vi "Teleop.vi"(10 "Match Info":T4={"Autonomous Elapsed Seconds"=0.0, "TeleOp Elapsed Seconds"=0.0, "Disabled Elapsed Seconds"=0.0, "Visited Autonomous"=FALSE, "Visited TeleOp"=FALSE, "Visited Disabled"=FALSE, "Autonomous Settings"={"Autonomous Style"=enum."Independent", "VI Refnum"=refnum}}, 11 "Call Context":T5) -> ()   [LabVIEW 2018]
doc: "This VI is called for each TeleOp packet received from the DS where the robot is not disabled. It is often used to read from the joysticks and update I/O or to update setpoints for timed control loops. It should complete and return within 20 milliseconds or it may miss DS packets."
uses:
  <vilib>/Rock Robotics/WPI/DriverStation/WPI_DriverStationDerivedRobotMode.ctl
  <vilib>/Rock Robotics/WPI/DriverStation/WPI_DriverStationMatch Info.ctl
  <vilib>/Rock Robotics/WPI/Solenoid/WPI_SolenoidValue.ctl
  <vilib>/Rock Robotics/WPI/ThirdParty/Phoenix-LabVIEW/Motor Controller/Controls/CTRE_Phoenix_MotorControl_ControlMode.ctl
  <vilib>/Rock Robotics/WPI/Utilities/WPI_GetSetVariantRefNum.vi
  <vilib>/Rock Robotics/WPI/Joystick/WPI_JoystickArcadeMapping.vi
  <vilib>/Rock Robotics/Network Tables/NT Write Boolean Array.vi
  <vilib>/Rock Robotics/Network Tables/NT Write Numeric Array.vi
  <vilib>/Rock Robotics/WPI/Solenoid/WPI_SolenoidSetEnum.vi
  <vilib>/Rock Robotics/WPI/ThirdParty/Phoenix-LabVIEW/Motor Controller/Get/CTRE_Phoenix_MotorController_GetSelectedSensorData.vi
  <vilib>/Rock Robotics/Network Tables/NT Read Boolean.vi
  Toolbox/Simple Limit Switch/Limits(Switch+Encoder).vi
  Toolbox/Simple Limit Switch/Limits(DoubleSwitch).vi
  Toolbox/Simple Limit Switch/Limits(SingleSwitch).vi
  <vilib>/Rock Robotics/Network Tables/NT Write Number.vi
panel:
  in  "Wrist Setpoints":dbl[](array[numeric])=[-144418.0, -146243.0, -22471.0, -33508.0, -1418.0, -92418.0, -108418.0, -72418.0, -202418.0]
  in  "Positive Feeder":dbl=1.0
  in  "Negative Feeder":dbl=-0.5
  out "Wrist  Encoder Value":i32
  out "Wrist Out":dbl
  out "Wrist PID Out":dbl
  out "Elevator Out":dbl
  out "Elevator PID Out":dbl
  in  "Outer Invert Motor Limit":bool
  in  "Outer Invert Encoder Limit":bool=TRUE
  in  "Outer Limit":dbl format="%#_13g"
  in  "Horse Invert Encoder Limit":bool=TRUE
  in  "Wrist Invert Encoder Limit":bool=TRUE
  in  "Elevator Invert Encoder Limit":bool=TRUE
  out "Horse Limit Switch":bool
  in  "Reset Horse Encoder":bool
  out "OuterStageSwitch":bool
  out "Wrist After Dangerzone":T1(ring)
  out "Elevator  After Dangerzone":T2(ring)
  in  "Elevator Auto":bool=TRUE
  in  "Elevator Output Range":cluster{"output high":dbl, "output low":dbl}={"output high"=0.66176470588, "output low"=-0.75}
  in  "Elevator PID Gains":T3={"proportional gain (Kc)"=-1e-05, "integral time (Ti, min)"=0.0, "derivative time (Td, min)"=0.0}
  in  "Elevator Setpoints":dbl[](array[numeric])=[-10000.0, -10000.0, -10000.0, 405000.0, 405000.0, -10000.0]
  in  "Wrist Auto":bool=TRUE
  in  "Wrist Output Range":cluster{"output high":dbl, "output low":dbl}={"output high"=0.5, "output low"=-0.5}
  in  "Wrist PID Gains":T3={"proportional gain (Kc)"=6e-05, "integral time (Ti, min)"=0.0, "derivative time (Td, min)"=0.0}
  in  "Wrist Invert Motor Limit":bool=TRUE
  out "Wrist Limit Switch":bool
  out "Elevator Limit Switch Top":bool
  in  "Elevator Invert Motor Limit":bool=TRUE
  in  "Intake Encoder Limit":dbl=-130000.0 format="%#_13g"
  in  "Intake Home Encoder Limit":dbl=-45000.0 format="%#_13g"
  in  "HorseDanger":i32=-600000
  in  "Horse  Encoder Limit":dbl=-190000.0 format="%#_13g"
  in  "Horse Invert Motor Limit":bool=TRUE
  out "Elevator Limit Switch":bool
  out "Elevator Encoder":i32=-47
  in  "Reset Elevator Encoder":bool
  out "Horse Encoder":i32
  in  "Reset Wrist Encoder":bool
  out "Intake Wrist Encoder":i32
  # "BETA POWER/DIRECTIONS\nElevator: Negative is up\nHorse: Negative is into robot\nOuter: Positive is down\nWrist: Negative is into robot"
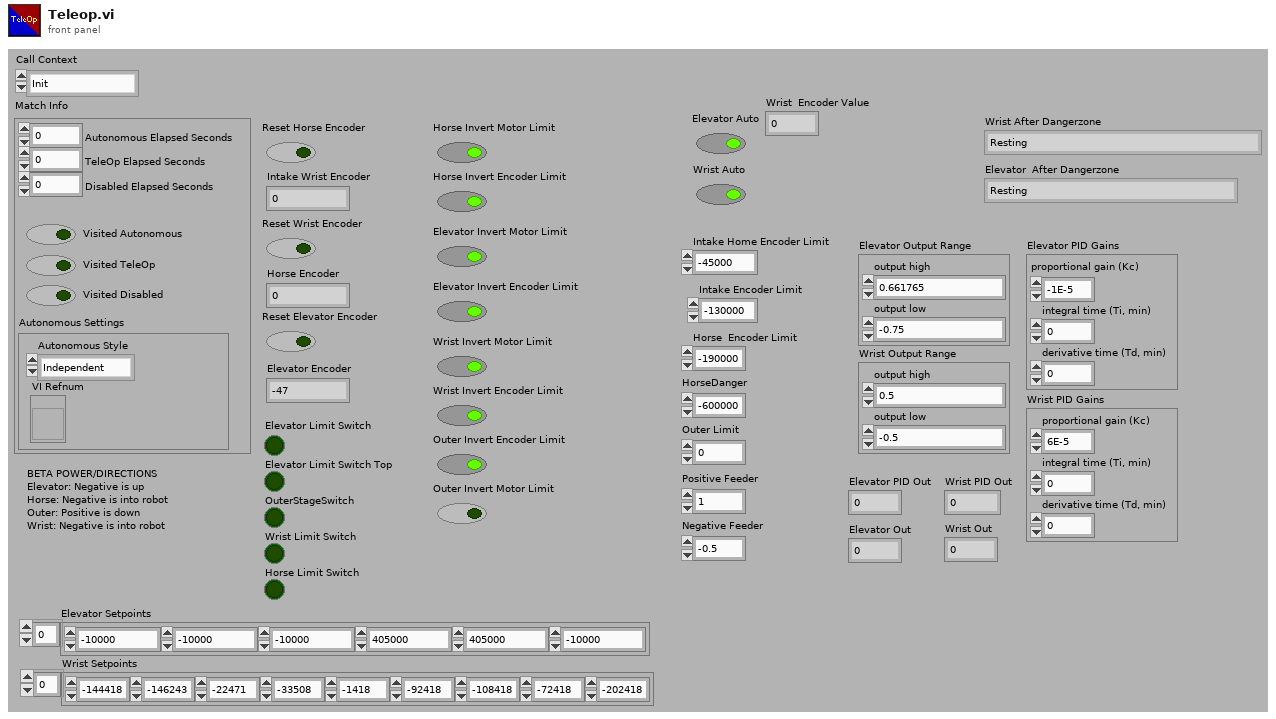
[diagram p1: front panel]
types:
  T1 = enum16{"Resting", "Hatch Ground Intake", "Hatch Place Low/Mid/CargoShip", "Hatch Place High", "Cargo Ground Intake", "Cargo Place Low/Mid", "Cargo Place High", "CargoShip Place Front", "CargoShip Place Back"}
  T2 = enum16{"Resting", "CargoShip Front", "CargoShip Back", "Cargo Mid", "Hatch Mid", "All High"}
  T3 = cluster{"proportional gain (Kc)":dbl, "integral time (Ti, min)":dbl, "derivative time (Td, min)":dbl}
  T4 = typedef "WPI_DriverStationMatch Info.ctl" = cluster{"Autonomous Elapsed Seconds":dbl, "TeleOp Elapsed Seconds":dbl, "Disabled Elapsed Seconds":dbl, "Visited Autonomous":bool, "Visited TeleOp":bool, "Visited Disabled":bool, "Autonomous Settings":cluster{"Autonomous Style":enum16{"Iterative", "Independent"}, "VI Refnum":refnum<vi>}}
  T5 = typedef "WPI_DriverStationDerivedRobotMode.ctl" = enum16{"Init", "Execute", "Stop"}
  T6 = typedef "WPI_SolenoidValue.ctl" = enum16{"Off", "On", "Forward", "Reverse"}
  T7 = enum16{"Intake Cargo", "Outtake Cargo", "Resting Cargo", "Intake Hatches", "Outtake Hatches", "Resting Hatches"}
  T8 = enum16{"Elevator Level 1", "Elevator Level 2", "Elevator Level 3"}
  T9 = typedef "CTRE_Phoenix_MotorControl_ControlMode.ctl" = u16
  T10 = cluster{"Intake Wheels Forwards":bool, "Elevator Shift":bool, "Intake Wheels Backwards":bool, "Drivetrain Shift":bool, "Elevator Outer Forwards":bool, "Elevator Outer Backwards":bool, "Hatch Telescope":bool, "Hatch Intake Clamp":bool, "Horse Drive Up":bool, "Horse Drive Down":bool, "Level 3 Climb":bool}
  T11 = typedef "WPI_JoystickDevRef.ctl" = cluster{"Device":T12}
  T12 = typedef "WPI_JoystickDeviceEnum.ctl" = enum16{"USB 0", "USB 1", "USB 2", "USB 3", "USB 4", "USB 5"}
  T13 = typedef "WPI_MotorControlDeviceRef.ctl" = cluster{"DeviceStatus":errorcluster, "Type":T14, "PWM":cluster{"PWM Channel":T15, "DeadBand":T16}, "CAN":cluster{"Device Number":u8, "SetOutput VI Ref":variant, "GetOutput VI Ref":variant, "Enable VI Ref":variant, "Disable VI Ref":variant, "Data":variant}, "Invert":bool, "DIO PWM":cluster{"PWM \"Enable\" Channel":T15, "DIOChannel":T17, "PWM Rate":dbl}}
  T14 = typedef "WPI_MotorControlType.ctl" = enum16{"PWM", "CAN", "DIO PWM"}
  T15 = typedef "FPGA_DIOPWMChannel.ctl" = enum8{"PWM 0", "PWM 1", "PWM 2", "PWM 3", "PWM 4", "PWM 5", "PWM 6", "PWM 7", "PWM 8", "PWM 9", "PWM MXP 0", "PWM MXP 1", "PWM MXP 2", "PWM MXP 3", "PWM MXP 4", "PWM MXP 5", "PWM MXP 6", "PWM MXP 7", "PWM MXP 8", "PWM MXP 9", "Invalid"}
  T16 = typedef "WPI_PWMDeadband.ctl" = cluster{"Name":string, "maxPositivePwm":i32, "minPositivePwm":i32, "centerPwm":i32, "maxNegativePwm":i32, "minNegativePwm":i32, "angularRange":u16}
  T17 = typedef "FPGA_DIOChannel.ctl" = enum8{"DIO 0", "DIO 1", "DIO 2", "DIO 3", "DIO 4", "DIO 5", "DIO 6", "DIO 7", "DIO 8", "DIO 9", "DIO MXP 0", "DIO MXP 1", "DIO MXP 2", "DIO MXP 3", "DIO MXP 4", "DIO MXP 5", "DIO MXP 6", "DIO MXP 7", "DIO MXP 8", "DIO MXP 9", "DIO MXP 10", "DIO MXP 11", "DIO MXP 12", "DIO MXP 13", "DIO MXP 14", "DIO MXP 15", "SPI Port CS1", "SPI Port CS2", "SPI Port CS3", "SPI Port MISO", "SPI Port MOSI", "Invalid"}
  T18 = typedef "WPI_SolenoidDevRef.ctl" = cluster{"DevStatus":errorcluster, "Pneumatics Control Module":u8, "Forward Solenoid Channel":T19, "Reverse Solenoid Channel":T19}
  T19 = typedef "WPI_SolenoidChannel.ctl" = enum8{"Solenoid 0", "Solenoid 1", "Solenoid 2", "Solenoid 3", "Solenoid 4", "Solenoid 5", "Solenoid 6", "Solenoid 7", "Invalid"}
  T20 = typedef "WPI_SwitchDevRef.ctl" = cluster{"DevStatus":errorcluster, "DIO Channel":T17, "CntIndex":T21, "Normally Closed":bool}
  T21 = typedef "FPGA_CounterCtrSystemIndex.ctl" = enum8{"Ctr 0", "Ctr 1", "Ctr 2", "Ctr 3", "Ctr 4", "Ctr 5", "Ctr 6", "Ctr 7", "Invalid"}
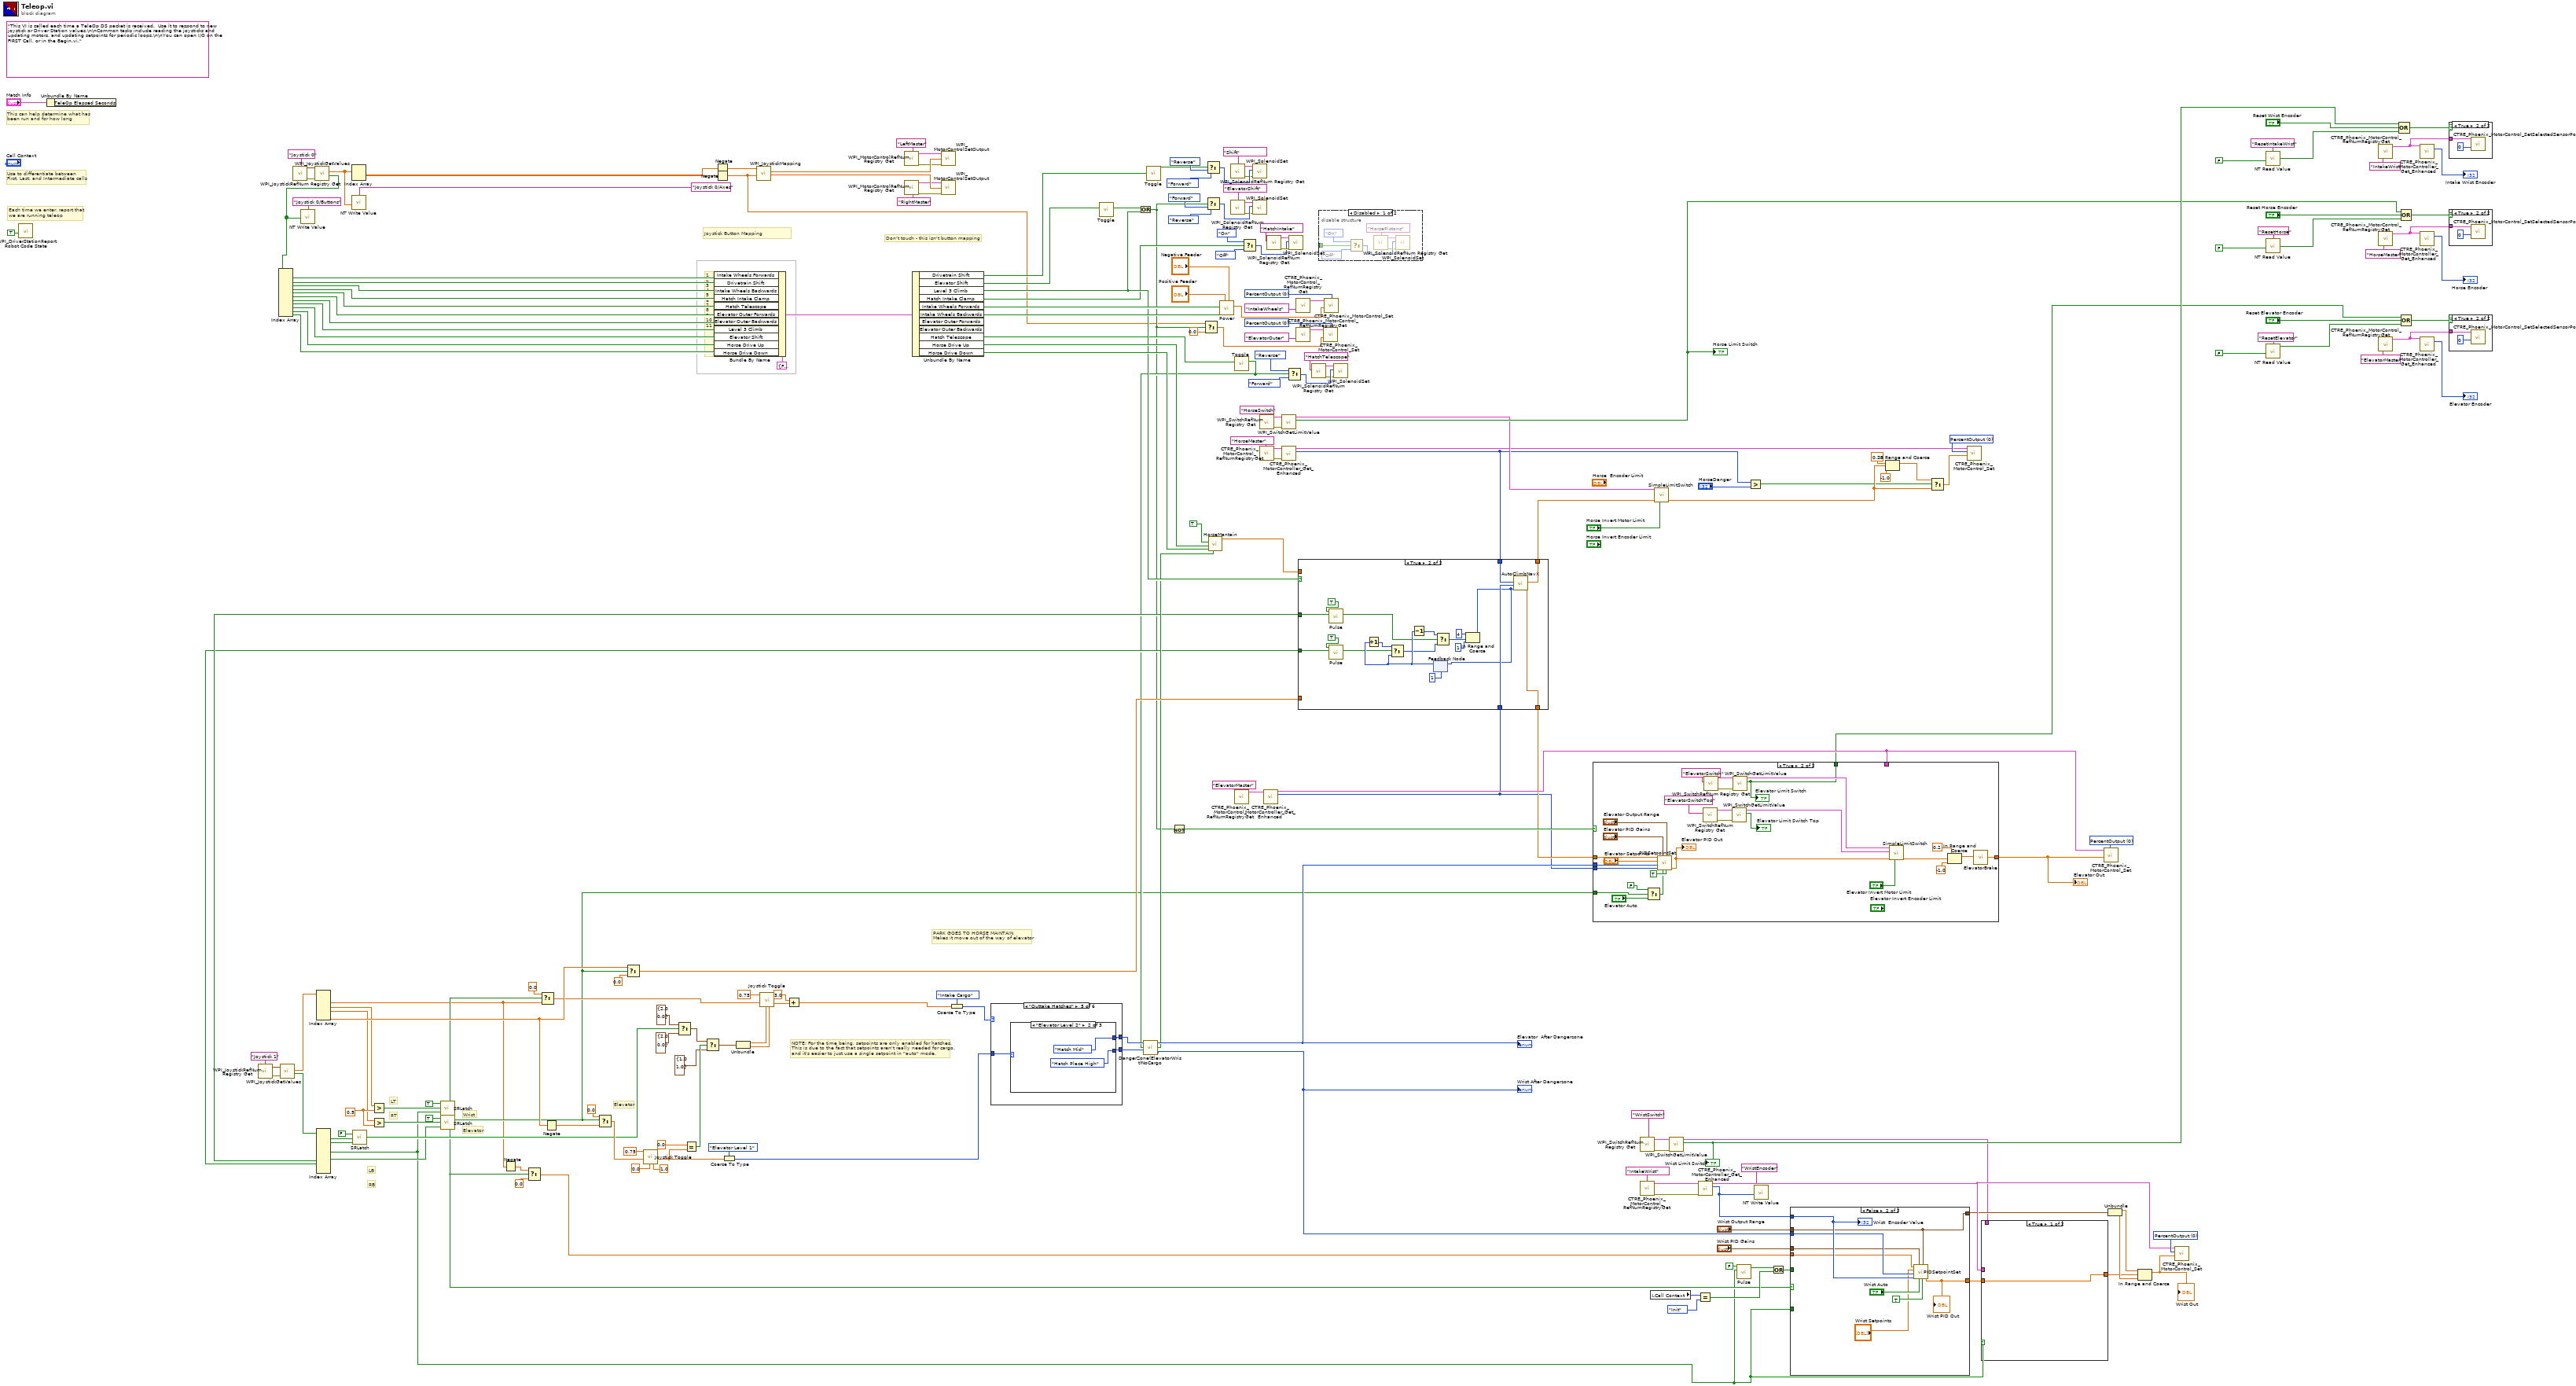
[diagram p0: block diagram]
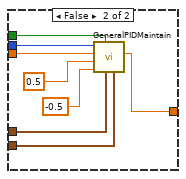
[diagram p3: hidden frame]
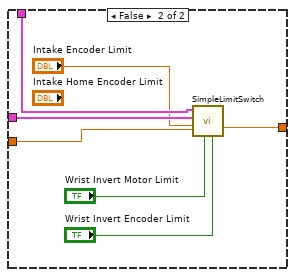
[diagram p4: hidden frame]
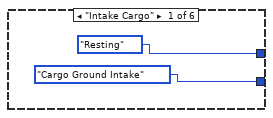
[diagram p6: hidden frame]
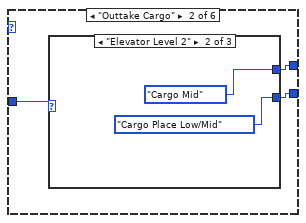
[diagram p7: hidden frame]
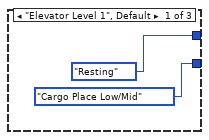
[diagram p8: hidden frame]
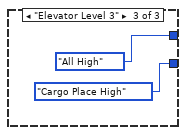
[diagram p9: hidden frame]
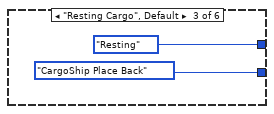
[diagram p10: hidden frame]
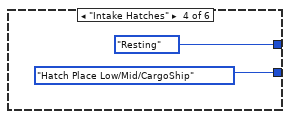
[diagram p11: hidden frame]
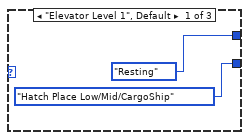
[diagram p12: hidden frame]
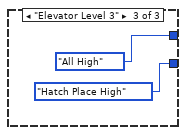
[diagram p13: hidden frame]
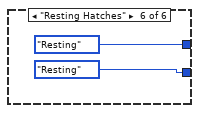
[diagram p14: hidden frame]
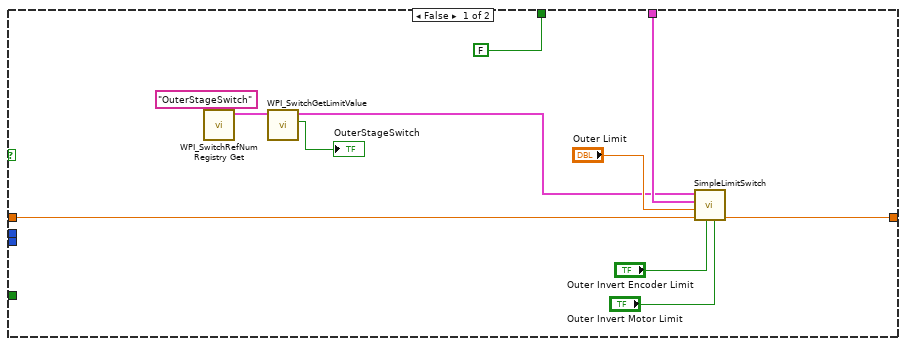
[diagram p16: hidden frame]
diagram:
  w35 = 0.5 ("t")
  w116 = T9 0 items=["PercentOutput"=0, "Position"=1, "Velocity"=2, "Current"=3, "Follower"=5, "MotionProfile"=6, "MotionMagic"=7, "MotionProfileArc"=10, "Disabled"=15] ("Control Mode")
  w120 = T9 0 items=["PercentOutput"=0, "Position"=1, "Velocity"=2, "Current"=3, "Follower"=5, "MotionProfile"=6, "MotionMagic"=7, "MotionProfileArc"=10, "Disabled"=15] ("Control Mode")
  w150 = T9 0 items=["PercentOutput"=0, "Position"=1, "Velocity"=2, "Current"=3, "Follower"=5, "MotionProfile"=6, "MotionMagic"=7, "MotionProfileArc"=10, "Disabled"=15] ("Control Mode")
  w159 = T9 0 items=["PercentOutput"=0, "Position"=1, "Velocity"=2, "Current"=3, "Follower"=5, "MotionProfile"=6, "MotionMagic"=7, "MotionProfileArc"=10, "Disabled"=15] ("Control Mode")
  w161 = T9 0 items=["PercentOutput"=0, "Position"=1, "Velocity"=2, "Current"=3, "Follower"=5, "MotionProfile"=6, "MotionMagic"=7, "MotionProfileArc"=10, "Disabled"=15] ("Control Mode")
  (unwired) "This VI is called each time a TeleOp DS packet is received.  Use it to respond to new joystick or Driver Station values.\n\nCommon tasks include reading the joysticks and updating motors, and updating setpoints for periodic loops.\n\nYou can open I/O on the FIRST Call, or in the Begin.vi."
  # "NOTE: For the time being, setpoints are only enabled for hatches.\nThis is due to the fact that setpoints aren't really needed for cargo, \nand it's easier to just use a single setpoint in \"auto\" mode."
  # "Elevator"
  # "Elevator"
  # "Wrist"
  # "LT"
  # "RT"
  # "RB"
  # "LB"
  # "Don't touch - this isn't button mapping"
  # "1\n2\n3\n4\n5\n6\n7\n8\n9\n10\n11"
  # "PARK GOES TO HORSE MAINTAIN\nMakes it move out of the way of elevator"
  # "Joystick Button Mapping"
  # "Each time we enter, report that\nwe are running teleop"
  # "Use to differentiate between\nFirst, Last, and Intermediate calls"
  # "This can help determine what has\nbeen run and for how long"
  n1 = call <vilib>:"WPI_DriverStationReport Robot Code State.vi"("TeleOp"=TRUE ("Autonomous")) -> ()  [unwired: 10 in, 1 out]
  n2 = Unbundle By Name("Match Info") -> ()  [unwired: 1 out]
  n3 = call <vilib>:"WPI_JoystickRefNum Registry Get.vi"("refnum name"="Joystick 1") -> ("error out"=w141:errorcluster, "JoystickDevRef"=w140:T11)  [unwired: 9 in]
  n4 = call <vilib>:"WPI_JoystickGetValues.vi"("error in (no error)"=w141, "JoystickDevRef"=w140) -> ("Buttons"=w127:bool[], "Axes"=w128:dbl[])  [unwired: 5 in, 3 out]
  n5 = call <vilib>:"WPI_JoystickRefNum Registry Get.vi"("refnum name"="Joystick 0") -> ("error out"=w188:errorcluster, "JoystickDevRef"=w221:T11)  [unwired: 1 in, 8 out]
  n6 = call <vilib>:"WPI_JoystickGetValues.vi"("error in (no error)"=w188, "JoystickDevRef"=w221) -> ("Buttons"=w185:bool[], "Axes"=w217:dbl[])  [unwired: 5 in, 3 out]
  n7 = Index Array(array=w185) -> (element #1=w205:bool, element #2=w215:bool, element #3=w214:bool, element #4=w213:bool, element #5=w212:bool, element #6=w211:bool, element #7=w210:bool, element #8=w209:bool, element #9=w208:bool, element #10=w207:bool, element #11=w206:bool)  [unwired: 11 in]
  n8 = call-poly <vilib>:"NT Write Value.vi"("Boolean Array"=w185, "Name"="Joystick 0/Buttons") -> ()  [unwired: 9 in, 1 out]
  n9 = Index Array(array=w128) -> (element #2=w10:dbl, element #3=w34:dbl, element #4=w33:dbl, element #6=w71:dbl)  [unwired: 6 in, 2 out]
  n10 = Index Array(array=w127) -> (element #1=w18:bool, element #4=w37:bool, element #5=w7:bool, element #6=w30:bool, element #7=w61:bool, element #8=w60:bool)  [unwired: 10 in, 4 out]
  n11 = Index Array(array=w217) -> (element #1=w164:dbl, element #2=w184:dbl)  [unwired: 2 in]
  n12 = call-poly <vilib>:"NT Write Value.vi"("Numeric Array"=w217, "Name"="Joystick 0/Axes") -> ()  [unwired: 9 in, 1 out]
  n13 = call "SRLatch.vi"("On"=w37, "Off"=w18, "Initial"=FALSE) -> ("Output"=w36:bool)
  n14 = Greater?(x=w34, y=w35) -> (0:w24:bool)
  n15 = Greater?(x=w33, y=w35) -> (0:w23:bool)
  n16 = call "SRLatch.vi"("On"=w7, "Off"=w24, "Initial"=TRUE) -> ("Output"=w12:bool)
  n17 = call "SRLatch.vi"("On"=w30, "Off"=w23, "Initial"=TRUE) -> ("Output"=w11:bool)
  n18 = Negate(x=w10) -> (-x=w73:dbl)
  n19 = Select(t=w73, s=w12, f=0.0) -> (s? t:f=w69:dbl)
  n20 = Select(t=0.0, s=w12, f=w10) -> (s? t:f=w65:dbl)
  n21 = Negate(x=w71) -> (-x=w64:dbl)
  n22 = Select(t=0.0, s=w11, f=w64) -> (s? t:f=w63:dbl)
  n23 = Select(t=w71, s=w11, f=0.0) -> (s? t:f=w70:dbl)
  n24 = call "Joystick Toggle.vi"("Max"=1.0, "Min"=0.0, "Value"=w63, "Range"=0.75) -> ("Output"=w89:dbl)  [unwired: 7 in]
  n25 = Select(t=cluster{"Range":dbl, "Range 2":dbl} {"Range"=2.0, "Range 2"=0.0}, s=w36, f=cluster{"Range":dbl, "Range 2":dbl} {"Range"=2.0, "Range 2"=0.0}) -> (s? t:f=w82:cluster{"Range":dbl, "Range 2":dbl})
  n26 = Equal?(x=0.0, y=w89) -> (x = y?=w81:bool)
  n27 = Select(t=w82, s=w81, f=cluster{"Range":dbl, "Range 2":dbl} {"Range"=1.0, "Range 2"=1.0}) -> (s? t:f=w83:cluster{"Range":dbl, "Range 2":dbl})
  n28 = Bundle By Name(cluster=T10 {"Intake Wheels Forwards"=FALSE, "Elevator Shift"=FALSE, "Intake Wheels Backwards"=FALSE, "Drivetrain Shift"=FALSE, "Elevator Outer Forwards"=FALSE, "Elevator Outer Backwards"=FALSE, "Hatch Telescope"=FALSE, "Hatch Intake Clamp"=FALSE, "Horse Drive Up"=FALSE, "Horse Drive Down"=FALSE, "Level 3 Climb"=FALSE} ("input cluster"), "Intake Wheels Forwards"=w205, "Drivetrain Shift"=w215, "Intake Wheels Backwards"=w214, "Hatch Intake Clamp"=w213, "Hatch Telescope"=w212, "Elevator Outer Forwards"=w211, "Elevator Outer Backwards"=w210, "Level 3 Climb"=w209, "Elevator Shift"=w208, "Horse Drive Up"=w207, "Horse Drive Down"=w206) -> (w204:T10)
  n29 = Negate(x=w164) -> (-x=w28:dbl)
  n30 = Negate(x=w184) -> (-x=w25:dbl)
  n31 = Coerce To Type(0:w89, 1:T8."Elevator Level 1") -> (2:w75:T8)
  n32 = Unbundle(w83) -> ("Range"=w85:dbl, "Range 2"=w84:dbl)
  n33 = call-poly <vilib>:"WPI_JoystickMapping.vi"("Y axis value"=w25, "X axis value"=w28) -> ("Right Motor Value"=w189:dbl, "Left Motor Value"=w190:dbl)  [unwired: 8 in]
  n34 = call "Joystick Toggle.vi"("Max"=w84, "Min"=w85, "Value"=w65, "Range"=0.75) -> ("Output"=w78:dbl)  [unwired: 7 in]
  n35 = Add(x=3.0 ("y"), y=w78) -> (x+y=w1:dbl)
  n36 = call <vilib>:"WPI_MotorControlRefNum Registry Get.vi"("refnum name"="LeftMaster") -> ("error out"=w138:errorcluster, "MotorControlDevRef"=w139:T13)  [unwired: 9 in]
  n37 = call <vilib>:"WPI_MotorControlRefNum Registry Get.vi"("refnum name"="RightMaster") -> ("error out"=w137:errorcluster, "MotorControlDevRef"=w136:T13)  [unwired: 9 in]
  n38 = Unbundle By Name(w204) -> ("Drivetrain Shift"=w183:bool, "Elevator Shift"=w96:bool, "Level 3 Climb"=w95:bool, "Hatch Intake Clamp"=w53:bool, "Intake Wheels Forwards"=w192:bool, "Intake Wheels Backwards"=w191:bool, "Hatch Telescope"=w51:bool, "Horse Drive Up"=w143:bool, "Horse Drive Down"=w144:bool)  [unwired: 2 out]
  n39 = call <vilib>:"WPI_MotorControlSetOutput.vi"("error in (no error)"=w138, "Output"=w190, "MotorControlDevRef"=w139) -> ()  [unwired: 6 in, 3 out]
  n40 = call <vilib>:"WPI_MotorControlSetOutput.vi"("error in (no error)"=w137, "Output"=w189, "MotorControlDevRef"=w136) -> ()  [unwired: 6 in, 3 out]
  n41 = Coerce To Type(0:w1, 1:T7."Intake Cargo") -> (2:w77:T7)
  n42 = case shown="\"Outtake Hatches\"" w77 {
    tunnel: [T1."Cargo Ground Intake" ("Wrist") w226 T1."CargoShip Place Back" ("Wrist") T1."Hatch Place Low/Mid/CargoShip" ("Wrist") w239 T1."Resting" ("Wrist")] -> w126
    tunnel: [T2."Resting" ("Elevator Level") w227 T2."Resting" ("Elevator Level") T2."Resting" ("Elevator Level") w240 T2."Resting" ("Elevator Level")] -> w124
    tunnel: w75 -> [_ w228 _ _ w241 _]
    frame "Intake Cargo" {
    }
    frame "Outtake Cargo" {
      n43 = case shown="\"Elevator Level 2\"" w228 {
        tunnel: [T2."Resting" ("Elevator Level") T2."Cargo Mid" ("Elevator Level") T2."All High" ("Elevator Level")] -> w227
        tunnel: [T1."Cargo Place Low/Mid" ("Wrist") T1."Cargo Place Low/Mid" ("Wrist") T1."Cargo Place High" ("Wrist")] -> w226
        frame "Elevator Level 1", Default {
        }
        frame "Elevator Level 2" {
        }
        frame "Elevator Level 3" {
        }
      }
    }
    frame "Resting Cargo", Default {
    }
    frame "Intake Hatches" {
    }
    frame "Outtake Hatches" {
      n44 = case shown="\"Elevator Level 2\"" w241 {
        tunnel: [T2."Resting" ("Elevator Level") T2."Hatch Mid" ("Elevator Level") T2."All High" ("Elevator Level")] -> w240
        tunnel: [T1."Hatch Place Low/Mid/CargoShip" ("Wrist") T1."Hatch Place High" ("Wrist") T1."Hatch Place High" ("Wrist")] -> w239
        frame "Elevator Level 1", Default {
        }
        frame "Elevator Level 2" {
        }
        frame "Elevator Level 3" {
        }
      }
    }
    frame "Resting Hatches" {
    }
  }
  n45 = call "Toggle.vi"("Input"=w96) -> ("Output"=w94:bool)  [unwired: 10 in]
  n46 = Or(x=w94, y=w95) -> (x .or. y?=w27:bool)
  n47 = call "Toggle.vi"("Input"=w183) -> ("Output"=w199:bool)  [unwired: 10 in]
  n48 = Not(x=w27) -> (.not. x?=w104:bool)
  n49 = Select(t=w25, s=w27, f=0.0) -> (s? t:f=w29:dbl)
  n50 = Select(t=WPI_SolenoidValue."Reverse" ("Value"), s=w199, f=WPI_SolenoidValue."Forward" ("Value")) -> (s? t:f=w198:T6)
  n51 = Select(t=WPI_SolenoidValue."Forward" ("Value"), s=w27, f=WPI_SolenoidValue."Reverse" ("Value")) -> (s? t:f=w197:T6)
  n52 = call "Power.vi"("Negative Power"="Negative Feeder", "Positive Power"="Positive Feeder", "Negative"=w191, "Positive"=w192) -> ("Output"=w160:dbl)  [unwired: 7 in]
  n53 = call <vilib>:"WPI_SolenoidRefNum Registry Get.vi"("refnum name"="Shift") -> ("error out"=w186:errorcluster, "SolenoidDevRef"=w202:T18)  [unwired: 9 in]
  n54 = call <vilib>:"WPI_SolenoidRefNum Registry Get.vi"("refnum name"="ElevatorShift") -> ("error out"=w187:errorcluster, "SolenoidDevRef"=w194:T18)  [unwired: 9 in]
  n55 = call "Toggle.vi"("Input"=w51) -> ("Output"=w38:bool)  [unwired: 10 in]
  n56 = call "DangerZone(ElevatorWrist)NoCargo.vi"("Wrist"=w126, "Telescope Out"=w38, "Level"=w124) -> ("Wrist"=w142:T1, "Park Horse"=w67:bool, "Level"=w125:T2)
  "Elevator  After Dangerzone" <- w125
  "Wrist After Dangerzone" <- w142
  n57 = call "HorseMantain.vi"("Park"=w67, "Negative"=w144, "Positive"=w143, "HorseToggle"=TRUE) -> ("Power"=w101:dbl)  [unwired: 7 in]
  n58 = call <vilib>:"CTRE_Phoenix_MotorControl_RefNumRegistryGet.vi"("refnum name"="ElevatorMaster") -> ("PhoenixMotorControlDevRef"=w108:T13)  [unwired: 9 in, 1 out]
  n59 = Select(t=WPI_SolenoidValue."On" ("Value"), s=w53, f=WPI_SolenoidValue."Off" ("Value")) -> (s? t:f=w54:T6)
  n60 = call-poly <vilib>:"WPI_SolenoidSet.vi"("error in (no error)"=w186, "Value"=w198, "SolenoidDevRef"=w202) -> ()  [unwired: 7 in, 2 out]
  n61 = call-poly <vilib>:"WPI_SolenoidSet.vi"("error in (no error)"=w187, "Value"=w197, "SolenoidDevRef"=w194) -> ()  [unwired: 7 in, 2 out]
  n62 = call <vilib>:"WPI_SwitchRefNum Registry Get.vi"("refnum name"="HorseSwitch") -> ("error out"=w123:errorcluster, "SwitchDevRef"=w106:T20)  [unwired: 9 in]
  n63 = call <vilib>:"CTRE_Phoenix_MotorControl_RefNumRegistryGet.vi"("refnum name"="HorseMaster") -> ("error out"=w68:errorcluster, "PhoenixMotorControlDevRef"=w109:T13)  [unwired: 9 in]
  n64 = call-poly <vilib>:"CTRE_Phoenix_MotorController_Get_Enhanced.vi"("PhoenixMotorControlDevRef"=w108) -> ("PhoenixMotorControlDevRef"=w107:T13, "Position (Raw Sensor Units)"=w97:i32)  [unwired: 11 in, 2 out]
  n65 = call <vilib>:"WPI_SolenoidRefNum Registry Get.vi"("refnum name"="HatchIntake") -> ("error out"=w58:errorcluster, "SolenoidDevRef"=w57:T18)  [unwired: 9 in]
  n66 = call <vilib>:"WPI_SwitchGetLimitValue.vi"("error in (no error)"=w123, "SwitchDevRef"=w106) -> ("Switch Pressed"=w133:bool, "SwitchDevRef"=w105:T20)  [unwired: 7 in, 1 out]
  "Horse Limit Switch" <- w133
  n67 = call-poly <vilib>:"CTRE_Phoenix_MotorController_Get_Enhanced.vi"("PhoenixMotorControlDevRef"=w109, "error in"=w68) -> ("PhoenixMotorControlDevRef"=w39:T13, "Position (Raw Sensor Units)"=w102:i32)  [unwired: 10 in, 2 out]
  n68 = Select(t=WPI_SolenoidValue."Reverse" ("Value"), s=w38, f=WPI_SolenoidValue."Forward" ("Value")) -> (s? t:f=w49:T6)
  n69 = call-poly <vilib>:"WPI_SolenoidSet.vi"("error in (no error)"=w58, "Value"=w54, "SolenoidDevRef"=w57) -> ()  [unwired: 7 in, 2 out]
  n70 = call <vilib>:"CTRE_Phoenix_MotorControl_RefNumRegistryGet.vi"("refnum name"="IntakeWheels") -> ("PhoenixMotorControlDevRef"=w162:T13)  [unwired: 9 in, 1 out]
  n71 = call <vilib>:"CTRE_Phoenix_MotorControl_RefNumRegistryGet.vi"("refnum name"="ElevatorOuter") -> ("PhoenixMotorControlDevRef"=w158:T13)  [unwired: 9 in, 1 out]
  n72 = case shown="True" w95 {
    tunnel: w102 -> [_ w270]
    tunnel: [w250 w269] -> w100
    tunnel: [w251 w268] -> w98
    tunnel: w70 -> [w251 _]
    tunnel: w101 -> [w250 _]
    tunnel: w97 -> [_ w267]
    tunnel: w61 -> [_ w257]
    tunnel: w60 -> [_ w254]
    frame False {
    }
    frame True {
      n73 = call "Pulse.vi"("Input"=w257, "Rising Edge?"=TRUE) -> ("Output"=w263:bool)  [unwired: 9 in]
      n74 = call "Pulse.vi"("Input"=w254, "Rising Edge?"=TRUE) -> ("Output"=w260:bool)  [unwired: 9 in]
      n75 = feedback #1(1) -> (w265:i32)
      n76 = Increment(x=w265) -> (x+1=w261:i32)
      n77 = Select(t=w261, s=w260, f=w265) -> (s? t:f=w262:i32)
      n78 = Decrement(x=w265) -> (x-1=w264:i32)
      n79 = Select(t=w264, s=w263, f=w262) -> (s? t:f=w266:i32)
      n80 = In Range and Coerce(upper limit=4, x=w266, lower limit=1) -> (coerced(x)=w252:i32)  [unwired: 1 out]
      n81 = feedback-in #1(w252) -> ()
      n82 = call "AutoClimbNavX.vi"("Stage"=w252, "Elevator Encoder"=w267, "Horse Encoder"=w270) -> ("Elevator Output"=w268:dbl, "Horse Output"=w269:dbl)  [unwired: 7 in]
    }
  }
  n83 = call <vilib>:"WPI_SolenoidRefNum Registry Get.vi"("refnum name"="HatchTelescope") -> ("error out"=w45:errorcluster, "SolenoidDevRef"=w46:T18)  [unwired: 9 in]
  n84 = disable-structure shown="Disabled" {
    disable-tunnel: _ -> [w271 _]
    frame Disabled {
      n85 = Select(t=WPI_SolenoidValue."On" ("Value"), s=w271, f=WPI_SolenoidValue."Off" ("Value")) -> (s? t:f=w277:T6)
      n86 = call <vilib>:"WPI_SolenoidRefNum Registry Get.vi"("refnum name"="HorsePistons") -> ("error out"=w272:errorcluster, "SolenoidDevRef"=w274:T18)  [unwired: 9 in]
      n87 = call-poly <vilib>:"WPI_SolenoidSet.vi"("error in (no error)"=w272, "Value"=w277, "SolenoidDevRef"=w274) -> ()  [unwired: 7 in, 2 out]
    }
    frame Enabled {
    }
  }
  n88 = call <vilib>:"CTRE_Phoenix_MotorControl_Set.vi"("Output"=w29, "Control Mode"=w159, "PhoenixMotorControlDevRef"=w158) -> ()  [unwired: 7 in, 2 out]
  n89 = call <vilib>:"CTRE_Phoenix_MotorControl_Set.vi"("Output"=w160, "Control Mode"=w161, "PhoenixMotorControlDevRef"=w162) -> ()  [unwired: 7 in, 2 out]
  n90 = call-poly <vilib>:"WPI_SolenoidSet.vi"("error in (no error)"=w45, "Value"=w49, "SolenoidDevRef"=w46) -> ()  [unwired: 7 in, 2 out]
  n91 = case shown="True" w104 {
    tunnel: w107 -> [w288 _]
    tunnel: w97 -> [_ w309]
    tunnel: w125 -> [_ w308]
    tunnel: w98 -> [w278 w305]
    tunnel: [w284 w303] -> w103
    tunnel: [FALSE ("Switch Pressed") w294] -> w99
    tunnel: w11 -> [_ w290]
    frame False {
      n92 = call <vilib>:"WPI_SwitchRefNum Registry Get.vi"("refnum name"="OuterStageSwitch") -> ("SwitchDevRef"=w283:T20)  [unwired: 9 in, 1 out]
      n93 = call <vilib>:"WPI_SwitchGetLimitValue.vi"("SwitchDevRef"=w283) -> ("Switch Pressed"=→"OuterStageSwitch":bool, "SwitchDevRef"=w280:T20)  [unwired: 8 in, 1 out]
      n94 = call-poly "SimpleLimitSwitch.vi"("Into Home Limit Is Pos (Encoder)"="Outer Invert Motor Limit", "Into Home Limit Is Pos (Motor)"="Outer Invert Encoder Limit", "Power In"=w278, "Encoder Limit"="Outer Limit", "Motor Ref"=w288, "Limit Switch Ref"=w280) -> ("Power Out"=w284:dbl)  [unwired: 5 in]
    }
    frame True {
      n95 = Select(t=FALSE ("Update"), s=w290, f="Elevator Auto") -> (s? t:f=w291:bool)
      n96 = call "PIDSetpointSet.vi"("Update"=TRUE, "Output Range"="Elevator Output Range", "Auto"=w291, "PID Gains"="Elevator PID Gains", "Encoder Position"=w309, "Level"=w308, "Setpoints"="Elevator Setpoints", "Manual Power"=w305) -> ("Power Out"=w307:dbl)  [unwired: 3 in]
      "Elevator PID Out" <- w307
      n97 = call <vilib>:"WPI_SwitchRefNum Registry Get.vi"("refnum name"="ElevatorSwitchTop") -> ("error out"=w296:errorcluster, "SwitchDevRef"=w298:T20)  [unwired: 9 in]
      n98 = call <vilib>:"WPI_SwitchRefNum Registry Get.vi"("refnum name"="ElevatorSwitch") -> ("error out"=w301:errorcluster, "SwitchDevRef"=w302:T20)  [unwired: 9 in]
      n99 = call <vilib>:"WPI_SwitchGetLimitValue.vi"("error in (no error)"=w296, "SwitchDevRef"=w298) -> ("Switch Pressed"=→"Elevator Limit Switch Top":bool, "SwitchDevRef"=w289:T20)  [unwired: 7 in, 1 out]
      n100 = call <vilib>:"WPI_SwitchGetLimitValue.vi"("error in (no error)"=w301, "SwitchDevRef"=w302) -> ("Switch Pressed"=w294:bool, "SwitchDevRef"=w299:T20)  [unwired: 7 in, 1 out]
      "Elevator Limit Switch" <- w294
      n101 = call-poly "SimpleLimitSwitch.vi"("Into Home Limit Is Pos"="Elevator Invert Motor Limit", "Power In"=w307, "2nd Limit Switch Ref"=w289, "Home Limit Switch Ref"=w299) -> ("Power Out"=w316:dbl)  [unwired: 7 in]
      n102 = In Range and Coerce(upper limit=0.2, x=w316, lower limit=-1.0) -> (coerced(x)=w304:dbl)  [unwired: 1 out]
      n103 = call "ElevatorBrake.vi"("Power In"=w304) -> ("Power Out"=w303:dbl)
    }
  }
  "Elevator Out" <- w103
  n104 = call <vilib>:"WPI_SwitchRefNum Registry Get.vi"("refnum name"="WristSwitch") -> ("error out"=w154:errorcluster, "SwitchDevRef"=w153:T20)  [unwired: 9 in]
  n105 = call <vilib>:"CTRE_Phoenix_MotorControl_RefNumRegistryGet.vi"("refnum name"="IntakeWrist") -> ("error out"=w6:errorcluster, "PhoenixMotorControlDevRef"=w151:T13)  [unwired: 9 in]
  n106 = local read "Call Context"() -> (w17:T5)
  n107 = call-poly "SimpleLimitSwitch.vi"("Into Home Limit Is Pos (Motor)"="Horse Invert Motor Limit", "Power In"=w100, "Limit Switch Ref"=w105) -> ("Power Out"=w112:dbl)  [unwired: 8 in]
  n108 = call <vilib>:"WPI_SwitchGetLimitValue.vi"("error in (no error)"=w154, "SwitchDevRef"=w153) -> ("Switch Pressed"=w145:bool, "SwitchDevRef"=w8:T20)  [unwired: 7 in, 1 out]
  "Wrist Limit Switch" <- w145
  n109 = call-poly <vilib>:"CTRE_Phoenix_MotorController_Get_Enhanced.vi"("PhoenixMotorControlDevRef"=w151, "error in"=w6) -> ("PhoenixMotorControlDevRef"=w149:T13, "Position (Raw Sensor Units)"=w5:i32)  [unwired: 10 in, 2 out]
  n110 = Equal?(x=w17, y=WPI_DriverStationDerivedRobotMode."Init") -> (x = y?=w13:bool)
  n111 = call "Pulse.vi"("Input"=w7, "Rising Edge?"=FALSE) -> ("Output"=w15:bool)  [unwired: 9 in]
  n112 = Greater?(x=w102, y="HorseDanger") -> (0:w110:bool)
  n113 = call-poly <vilib>:"NT Write Value.vi"("Numeric"=w5, "Name"="WristEncoder") -> ()  [unwired: 9 in, 1 out]
  n114 = Or(x=w15, y=w13) -> (x .or. y?=w14:bool)
  n115 = case shown="False" w12 {
    tunnel: w5 -> [w321 w341]
    tunnel: w142 -> [_ w340]
    tunnel: [w322 w339] -> w129
    tunnel: w69 -> [w323 w337]
    tunnel: [w319 w334] -> w43
    tunnel: "Wrist PID Gains" -> [w320 w335]
    tunnel: "Wrist Output Range" -> [w319 w334]
    tunnel: w7 -> [w318 _]
    tunnel: w14 -> [w317 _]
    frame True {
      n116 = case shown="True" w318 {
        tunnel: w323 -> [w324 w332]
        tunnel: [w324 w331] -> w322
        tunnel: w321 -> [_ w330]
        tunnel: w320 -> [_ w327]
        tunnel: w319 -> [_ w326]
        tunnel: w317 -> [_ w325]
        frame True {
        }
        frame False {
          n117 = call "GeneralPIDMaintain.vi"("PID gains"=w327, "Output Range"=w326, "Initialize"=w325, "Lower Power Limit"=-0.5, "Upper Power Limit"=0.5, "Power"=w332, "Encoder Position"=w330) -> ("Power Out"=w331:dbl)  [unwired: 4 in]
        }
      }
    }
    frame False {
      n118 = call "PIDSetpointSet.vi"("Update"=TRUE, "Output Range"=w334, "Auto"="Wrist Auto", "PID Gains"=w335, "Encoder Position"=w341, "Level"=w340, "Setpoints"="Wrist Setpoints", "Manual Power"=w337) -> ("Power Out"=w339:dbl)  [unwired: 3 in]
      "Wrist PID Out" <- w339
      "Wrist  Encoder Value" <- w341
    }
  }
  n119 = In Range and Coerce(upper limit=0.25, x=w112, lower limit=-1.0) -> (coerced(x)=w113:dbl)  [unwired: 1 out]
  n120 = Select(t=w113, s=w110, f=w112) -> (s? t:f=w111:dbl)
  n121 = call <vilib>:"CTRE_Phoenix_MotorControl_Set.vi"("Output"=w111, "Control Mode"=w120, "PhoenixMotorControlDevRef"=w39) -> ()  [unwired: 7 in, 2 out]
  n122 = case shown="True" w7 {
    tunnel: [w342 w349] -> w40
    tunnel: w149 -> [_ w348]
    tunnel: w129 -> [w342 w345]
    tunnel: w8 -> [_ w344]
    frame True {
    }
    frame False {
      n123 = call-poly "SimpleLimitSwitch.vi"("Into Home Limit Is Pos (Encoder)"="Wrist Invert Encoder Limit", "Into Home Limit Is Pos (Motor)"="Wrist Invert Motor Limit", "Power In"=w345, "Encoder Limit"="Intake Encoder Limit", "Motor Ref"=w348, "Limit Switch Ref"=w344) -> ("Power Out"=w349:dbl)  [unwired: 5 in]
    }
  }
  n124 = call <vilib>:"CTRE_Phoenix_MotorControl_Set.vi"("Output"=w103, "Control Mode"=w116, "PhoenixMotorControlDevRef"=w107) -> ()  [unwired: 7 in, 2 out]
  n125 = Unbundle(w43) -> ("output high"=w42:dbl, "output low"=w41:dbl)
  n126 = In Range and Coerce(upper limit=w42, x=w40, lower limit=w41) -> (coerced(x)=w44:dbl)  [unwired: 1 out]
  "Wrist Out" <- w44
  n127 = call <vilib>:"CTRE_Phoenix_MotorControl_Set.vi"("Output"=w44, "Control Mode"=w150, "PhoenixMotorControlDevRef"=w149) -> ()  [unwired: 7 in, 2 out]
  n128 = call-poly <vilib>:"NT Read Value.vi"("Default Value"=FALSE, "Name"="ResetIntakeWrist") -> ("Boolean"=w172:bool)  [unwired: 8 in, 1 out]
  n129 = call-poly <vilib>:"NT Read Value.vi"("Default Value"=FALSE, "Name"="ResetHorse") -> ("Boolean"=w169:bool)  [unwired: 8 in, 1 out]
  n130 = call-poly <vilib>:"NT Read Value.vi"("Default Value"=FALSE, "Name"="ResetElevator") -> ("Boolean"=w148:bool)  [unwired: 8 in, 1 out]
  n131 = call <vilib>:"CTRE_Phoenix_MotorControl_RefNumRegistryGet.vi"("refnum name"="IntakeWrist") -> ("PhoenixMotorControlDevRef"=w180:T13)  [unwired: 9 in, 1 out]
  n132 = call <vilib>:"CTRE_Phoenix_MotorControl_RefNumRegistryGet.vi"("refnum name"="HorseMaster") -> ("PhoenixMotorControlDevRef"=w179:T13)  [unwired: 9 in, 1 out]
  n133 = call <vilib>:"CTRE_Phoenix_MotorControl_RefNumRegistryGet.vi"("refnum name"="ElevatorMaster") -> ("PhoenixMotorControlDevRef"=w174:T13)  [unwired: 9 in, 1 out]
  n134 = Compound Arithmetic op=OR(w145, "Reset Wrist Encoder", w172) -> (w130:bool)
  n135 = Compound Arithmetic op=OR(w133, "Reset Horse Encoder", w169) -> (w131:bool)
  n136 = Compound Arithmetic op=OR(w99, "Reset Elevator Encoder", w148) -> (w132:bool)
  n137 = call-poly <vilib>:"CTRE_Phoenix_MotorController_Get_Enhanced.vi"("PhoenixMotorControlDevRef"=w180) -> ("Position (Raw Sensor Units)"=→"Intake Wrist Encoder":i32)  [unwired: 11 in, 3 out]
  n138 = call-poly <vilib>:"CTRE_Phoenix_MotorController_Get_Enhanced.vi"("PhoenixMotorControlDevRef"=w179) -> ("Position (Raw Sensor Units)"=→"Horse Encoder":i32)  [unwired: 11 in, 3 out]
  n139 = call-poly <vilib>:"CTRE_Phoenix_MotorController_Get_Enhanced.vi"("PhoenixMotorControlDevRef"=w174) -> ("Position (Raw Sensor Units)"=→"Elevator Encoder":i32)  [unwired: 11 in, 3 out]
  n140 = case shown="True" w130 {
    tunnel: w180 -> [_ w351]
    frame False {
    }
    frame True {
      n141 = call <vilib>:"CTRE_Phoenix_MotorControl_SetSelectedSensorPosition.vi"("New Sensor Position"=0, "PhoenixMotorControlDevRef"=w351) -> ()  [unwired: 8 in, 2 out]
    }
  }
  n142 = case shown="True" w131 {
    tunnel: w179 -> [_ w353]
    frame False {
    }
    frame True {
      n143 = call <vilib>:"CTRE_Phoenix_MotorControl_SetSelectedSensorPosition.vi"("New Sensor Position"=0, "PhoenixMotorControlDevRef"=w353) -> ()  [unwired: 8 in, 2 out]
    }
  }
  n144 = case shown="True" w132 {
    tunnel: w174 -> [_ w355]
    frame False {
    }
    frame True {
      n145 = call <vilib>:"CTRE_Phoenix_MotorControl_SetSelectedSensorPosition.vi"("New Sensor Position"=0, "PhoenixMotorControlDevRef"=w355) -> ()  [unwired: 8 in, 2 out]
    }
  }
